vi "ex_subFileRead.vi"(0 "file path in":path, 1 "First Column is Time Channel":bool, 2 "file dialog?":bool, 3 "relative time?":bool, 4 "Attempt to Read Generic Text Files":bool, 5 "samples to read":i32=1, 6 "error in (no error)":errorcluster, 7 "delimiter":string="\t", 8 "First Row is Channel Names":bool, 9 "Decimal point":enum32{". (dot)", ", (comma)"}(radio), 10 "static path in":path, 11 "override samples":bool, 13 "Enable":bool=TRUE, 14 "Start Row":i32=1, 15 "storage_format":T6, 18 "single values":bool, 19 "Lock file":bool, 21 "Reset":bool) -> (12 "Description":string, 16 "Comment":string, 17 "EOF?":bool, 20 "file path out":path, 22 "Signals":dynamicdata(waveform), 26 "error out":errorcluster)   [LabVIEW 2020]
uses:
  <vilib>/express/express input/ExFileReadBlock.llb/ex_ReadFileGenericParams.ctl
  <vilib>/express/express shared/ExFile.llb/ex_FileFormats.ctl
  <vilib>/Platform/express/TDMExpress.llb/ex_readInfoTDM.ctl
  <vilib>/Platform/express/TDMExpress.llb/ex_readChannelInfo.ctl
  <vilib>/express/express shared/ExFile.llb/ex_TdmData.ctl
  <vilib>/express/express shared/ExFile.llb/ex_TdmProperty.ctl
  <vilib>/express/express shared/ex_EditUserDefinedProperties/usiDataType.ctl
panel:
  in  "Boolean":bool
  in  "read info":T1
  in  "read info in":T1
  in  "Lock file 2":bool
  out "previous path":path
  in  "Generic Params":T7
  in  "1st":bool
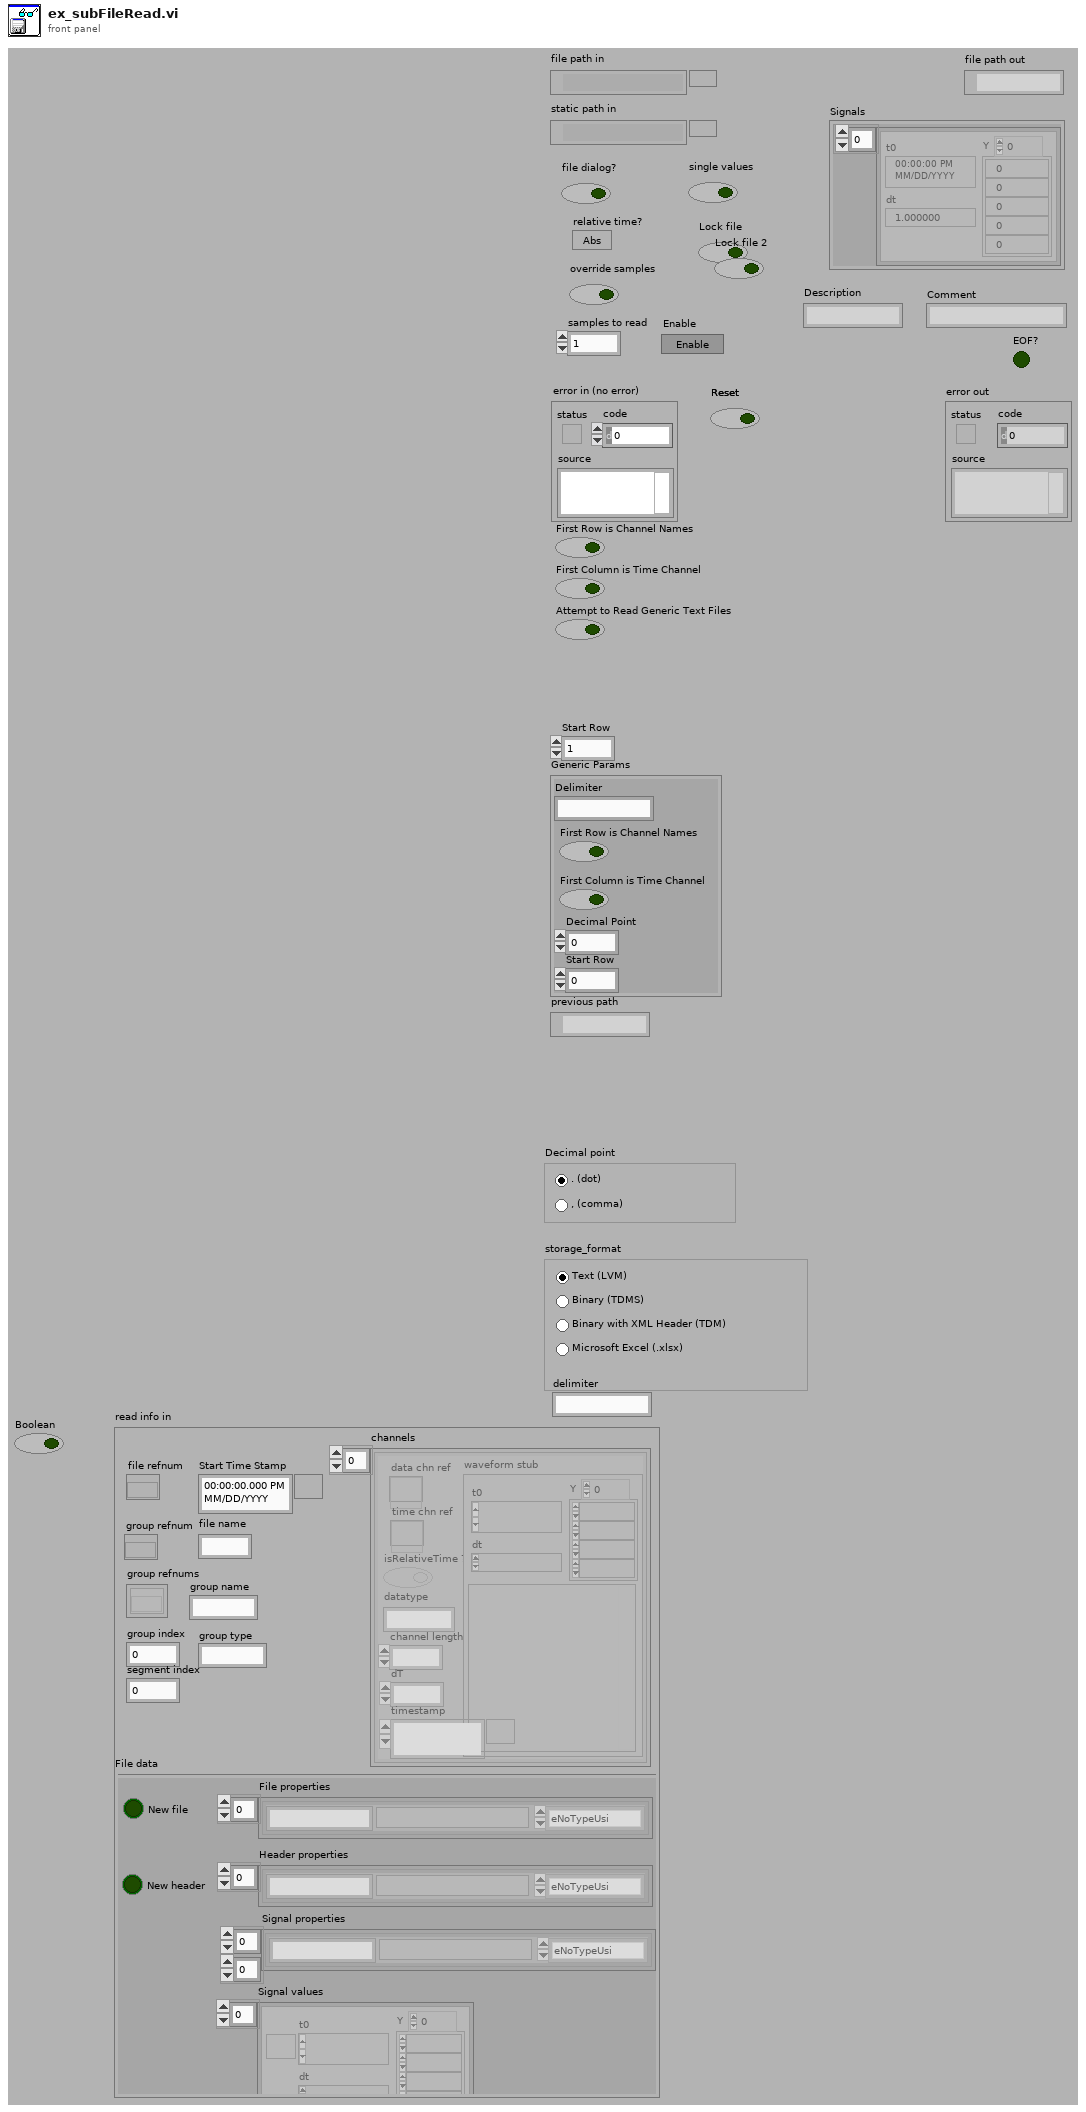
[diagram p1: front panel]
types:
  T1 = typedef "ex_readInfoTDM.ctl" = cluster{"file refnum":refnum<k20>, "group refnum":refnum<k20>, "group name":string, "group type":string, "Start Time Stamp":timestamp, "group index":u32, "group refnums":refnum<k20>[], "file name":string, "segment index":u32, "channels":T2[], "File data":T3}
  T2 = typedef "ex_readChannelInfo.ctl" = cluster{"data chn ref":refnum<k20>, "time chn ref":refnum<k20>, "isRelativeTime ?":bool, "channel length":u32, "dT":dbl, "waveform stub":waveform(dbl), "datatype":string, "timestamp":timestamp}
  T3 = typedef "ex_TdmData.ctl" = cluster{"New file":bool, "New header":bool, "File properties":T4[], "Header properties":T4[], "Signal properties":T4[][], "Signal values":waveform(dbl)[]}
  T4 = typedef "ex_TdmProperty.ctl" = cluster{"Name":string, "Type":T5, "Value":variant}
  T5 = typedef "usiDataType.ctl" = enum16{"eNoTypeUsi", "eInt8Usi", "eInt16Usi", "eInt32Usi", "eInt64Usi", "eUInt8Usi", "eUInt16Usi", "eUInt32Usi", "eUInt64Usi", "eFloat32Usi", "eFloat64Usi", "- 0", "- 1", "- 2", "- 3", "- 4", "- 5", "- 6", "- 7", "- 8", "- 9", "eString8Usi", "eString16Usi", "eStringUsi", "eEnumUsi", "- 10", "- 11", "- 12", "- 13", "- 14", "eTimeUsi", "- 15", "- 16", "- 17", "- 18", "- 19", "- 20", "- 21", "- 22", "- 23", "eInstanceUsi", "eStoreUsi"}
  T6 = typedef "ex_FileFormats.ctl" = enum32{"lvm", "tdm", "tdms", "xlsx"}
  T7 = typedef "ex_ReadFileGenericParams.ctl" = cluster{"Delimiter":string, "First Row is Channel Names":bool, "First Column is Time Channel":bool, "Decimal Point":i32, "Start Row":i32}
  T8 = typedef "ex_ReadFileParams.ctl" = cluster{"include col headings?":bool, "x_columns":u16, "col headings always?":bool, "time preference":u16, "hide col headings":bool}
  T9 = typedef "ex_AllChanInfo.ctl" = cluster{"No.Samples":i32, "Timestamp":timestamp, "X Dimension":string, "Y Dimension":string, "X0":timestamp, "Delta X":dbl, "Signal Name":string, "X Unit Label":string, "Y Unit Label":string}
  T10 = typedef "ex_FileReference.ctl" = cluster{"file ref":refnum<file>, "file size (bytes:0)":i32, "read pointer (bytes:0)":i32, "chunk size (bytes:65000)":i32}
  T11 = cluster{"chunk in":string, "file_params":T8, "delimiter":string, "optional info":cluster{"description":string, "operator":string, "project":string}, "Generic Header In":string[], "channel info":T9[], "read segment header in":bool, "# of samples read (in)":u32, "# of samples to read":i32, "# of samples in Channel Group":i32, "file refs in":T10, "origin timestamp":timestamp, "Is generic text file":bool, "Decimal Separator":string}
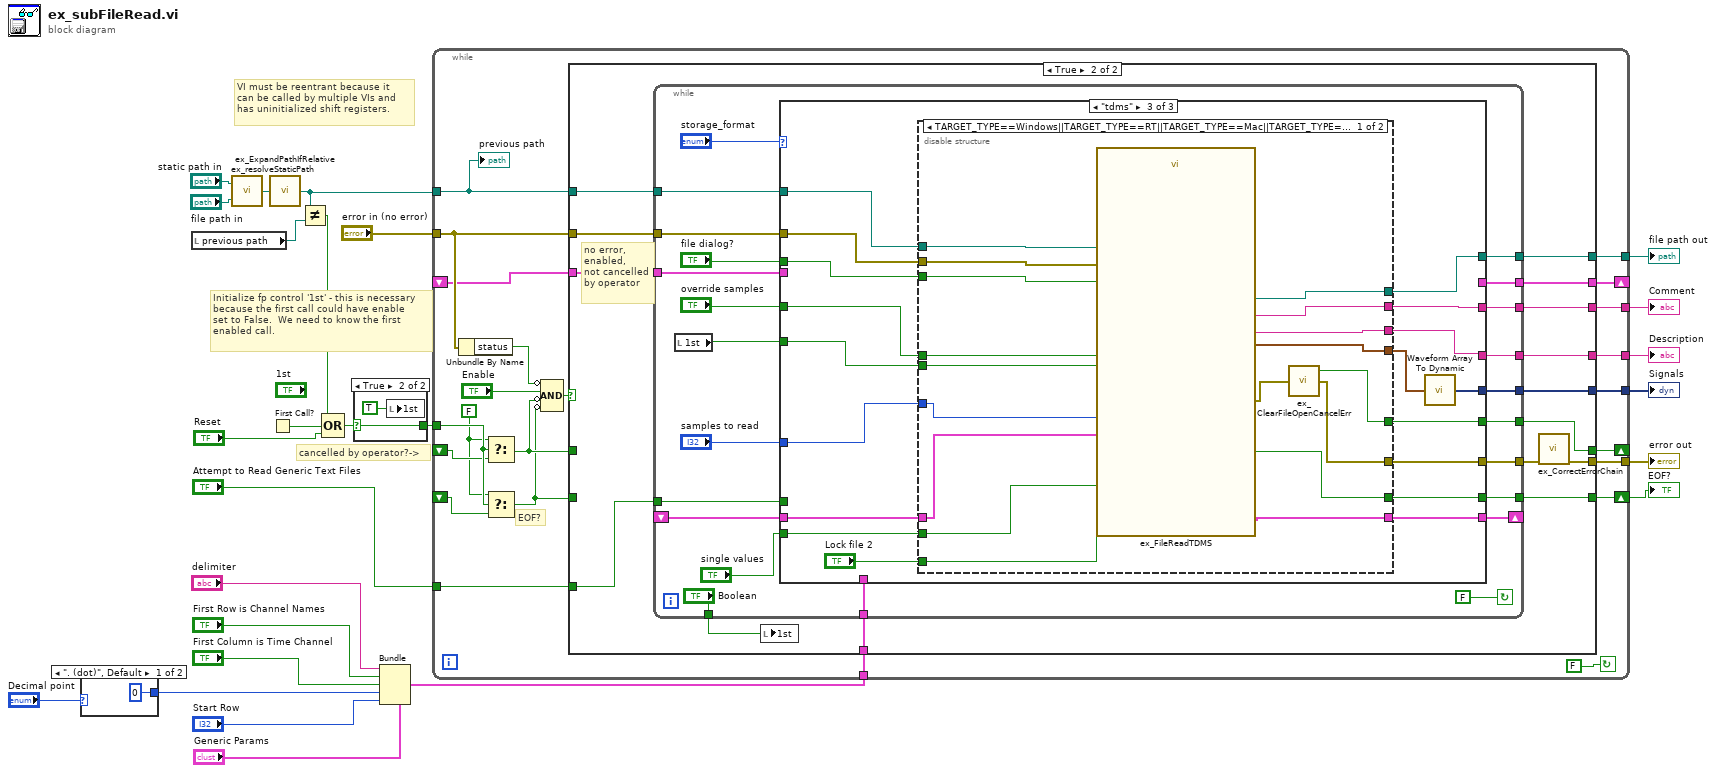
[diagram p0: block diagram]
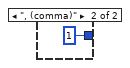
[diagram p2: hidden frame]
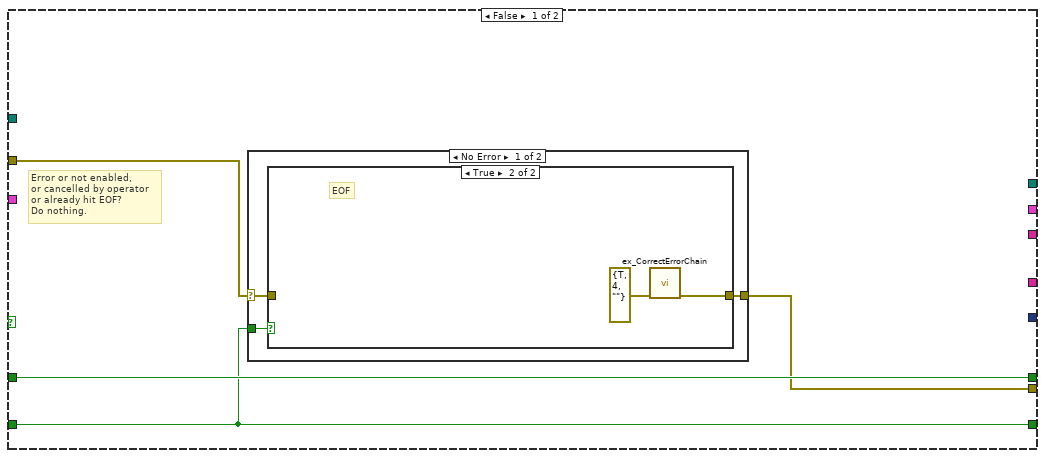
[diagram p3: hidden frame]
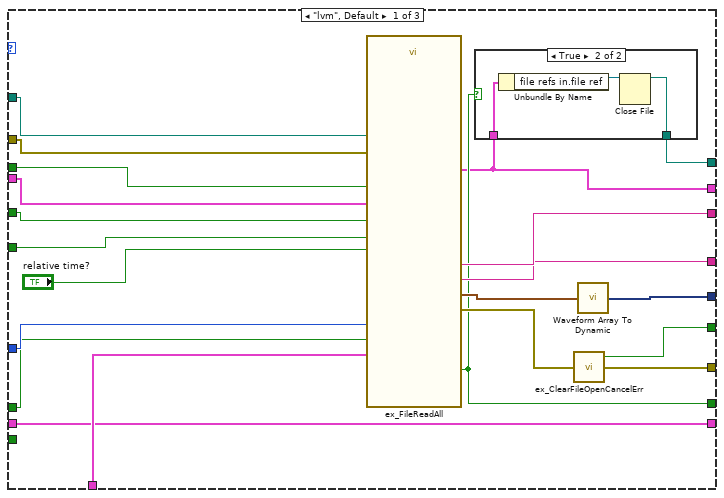
[diagram p6: hidden frame]
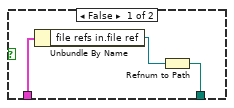
[diagram p7: hidden frame]
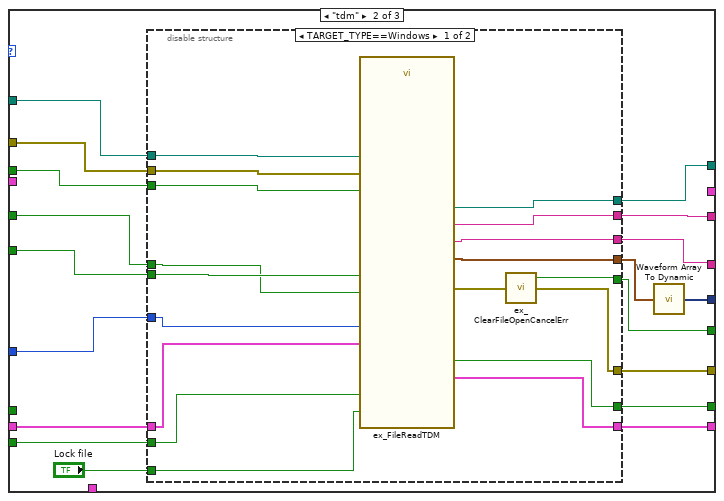
[diagram p8: hidden frame]
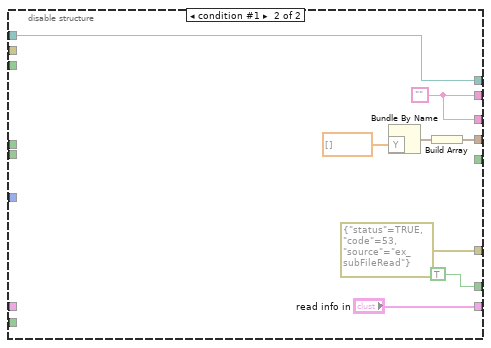
[diagram p9: hidden frame]
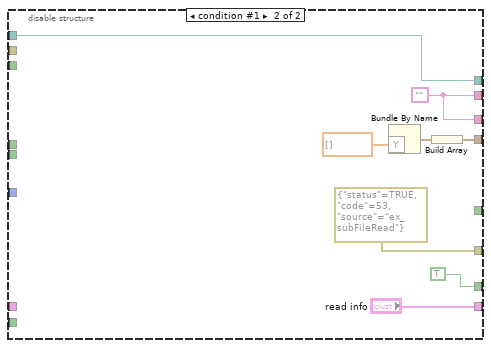
[diagram p10: hidden frame]
diagram:
  # "cancelled by operator?->"
  # "Initialize fp control '1st' - this is necessary \nbecause the first call could have enable \nset to False.  We need to know the first\nenabled call."
  # "VI must be reentrant because it \ncan be called by multiple VIs and \nhas uninitialized shift registers."
  n1 = case shown="\". (dot)\", Default" "Decimal point" {
    tunnel: [0 1] -> w3
    frame ". (dot)", Default {
    }
    frame ", (comma)" {
    }
  }
  n2 = local read "previous path"() -> (w14:path)
  n3 = call <vilib>:"ex_resolveStaticPath.vi"("file path in"="file path in", "static path in"="static path in") -> ("Path"=w15:path)
  n4 = First Call?() -> (First Call?: T/F=w26:bool)
  n5 = call <vilib>:"ex_ExpandPathIfRelative.vi"("Path"=w15) -> ("Expanded path"=w2:path)  [unwired: 4 out]
  n6 = Not Equal?(x=w2, y=w14) -> (x != y?=w12:bool)
  n7 = Compound Arithmetic op=OR(w12, w26, "Reset") -> (w13:bool)
  n8 = case shown="True" w13 {
    selector: w13 -> [w29 w30]
    tunnel: [w29 w30] -> w25
    frame False {
    }
    frame True {
      n9 = local write "1st"(TRUE ("1st")) -> ()
    }
  }
  n10 = Bundle(cluster="Generic Params", "Delimiter"="delimiter", "First Row is Channel Names"="First Row is Channel Names", "First Column is Time Channel"="First Column is Time Channel", "Decimal Point"=w3, "Start Row"="Start Row") -> (w18:T7)
  n11 = while {
    tunnel: [w54] -> w11
    tunnel: w25 -> [w40]
    tunnel: "error in (no error)" -> [w53]
    shift-right: [w49] -> _
    shift-left: _ -> [w39]
    tunnel: "Attempt to Read Generic Text Files" -> [w48]
    tunnel: w18 -> [w47]
    tunnel: w2 -> [w46]
    tunnel: [w45] -> w10
    tunnel: [w44] -> w9
    tunnel: [w43] -> w8
    tunnel: [w42] -> w7
    shift-right: [w41] -> w6
    shift-left: _ -> [w37]
    shift-right: [w32] -> _
    shift-left: _ -> [w33]
    stop <- FALSE continue-if-true
    w38 = FALSE ("operator cancelled?")
    # "EOF?"
    n12 = Unbundle By Name(w53) -> ("status"=w35:bool)
    n13 = Select(t=w38, s=w40, f=w39) -> (s? t:f=w36:bool)
    n14 = Select(t=w38, s=w40, f=w37) -> (s? t:f=w34:bool)
    n15 = Compound Arithmetic op=AND(invert w35, "Enable", invert w36, invert w34) -> (w50:bool)
    n16 = case shown="True" w50 {
      tunnel: [w56 w73] -> w54
      tunnel: w53 -> [w57 w80]
      tunnel: [w58 w78] -> w49
      tunnel: w36 -> [w58 _]
      tunnel: w48 -> [_ w77]
      tunnel: w47 -> [_ w76]
      tunnel: w46 -> [_ w75]
      tunnel: [_ w72] -> w45
      tunnel: [_ w71] -> w44
      tunnel: [_ w70] -> w43
      tunnel: [_ w69] -> w42
      tunnel: [w55 w68] -> w41
      tunnel: w34 -> [w55 _]
      tunnel: w33 -> [_ w67]
      tunnel: [_ w66] -> w32
      frame False {
        # "Error or not enabled,\nor cancelled by operator\nor already hit EOF?\nDo nothing."
        n17 = case shown="No Error" w57 {
          selector: w57 -> [w59 w65]
          tunnel: [w60 w65] -> w56
          tunnel: w55 -> [w61 _]
          frame No Error {
            n18 = case shown="True" w61 {
              tunnel: [w62 w64] -> w60
              tunnel: w59 -> [w62 _]
              frame False {
                # "not EOF"
              }
              frame True {
                # "EOF"
                n19 = call <vilib>:"ex_CorrectErrorChain.vi"("error in (no error)"=errorcluster {"status"=TRUE, "code"=4, "source"=""}) -> ("error out"=w64:errorcluster)  [unwired: 1 in, 9 out]
              }
            }
          }
          frame Error {
          }
        }
      }
      frame True {
        # "no error,\nenabled,\nnot cancelled\nby operator"
        n20 = while {
          tunnel: [w100] -> w74
          tunnel: w80 -> [w103]
          tunnel: ["Boolean"] -> w79
          tunnel: [w99] -> w78
          tunnel: w77 -> [w98]
          tunnel: w76 -> [w97]
          tunnel: w75 -> [w96]
          tunnel: [w95] -> w72
          tunnel: [w94] -> w71
          tunnel: [w93] -> w70
          tunnel: [w92] -> w69
          tunnel: [w91] -> w68
          tunnel: w67 -> [w86]
          tunnel: [w85] -> w66
          shift-right: [w82] -> _
          shift-left: _ -> [w83]
          stop <- FALSE continue-if-true
          n21 = local read "1st"() -> (w89:bool)
          n22 = case shown="\"tdms\"" "storage_format" {
            tunnel: w103 -> [w120 w147 w191]
            tunnel: [w124 w142 w186] -> w100
            tunnel: [w123 w131 w175] -> w99
            tunnel: w98 -> [w115 _ _]
            tunnel: w97 -> [w110 _ _]
            tunnel: w96 -> [w121 w148 w192]
            tunnel: [w105 w145 w189] -> w95
            tunnel: [w112 w144 w188] -> w94
            tunnel: [w111 w143 w187] -> w93
            tunnel: [w122 w133 w177] -> w92
            tunnel: [w107 w140 w184] -> w91
            tunnel: w89 -> [w118 w137 w181]
            tunnel: "samples to read" -> [w116 w141 w185]
            tunnel: "override samples" -> [w119 w136 w180]
            tunnel: w86 -> [w109 _ _]
            tunnel: [w106 _ _] -> w85
            tunnel: "file dialog?" -> [w108 w146 w190]
            tunnel: w83 -> [w104 w139 w183]
            tunnel: [w104 w138 w182] -> w82
            tunnel: "single values" -> [_ w135 w179]
            frame "lvm", Default {
              n23 = call <vilib>:"ex_FileReadAll.vi"("Parsing Data and Options In"=w109, "Generic File Read Parameters"=w110, "Attempt to Read Generic Text Files"=w115, "first_time?"=w118, "file dialog?"=w108, "error in (no error)"=w120, "file path in"=w121, "use specified sample size"=w119, "Samples to read"=w116, "relative time?"="relative time?") -> ("end-of-file?"=w107:bool, "Parsing Data and Options Out"=w106:T11, "Signals"=w113:waveform(dbl)[], "Description"=w111:string, "Comment"=w112:string, "error out"=w114:errorcluster)  [unwired: 4 out]
              n24 = case shown="True" w107 {
                tunnel: w106 -> [w127 w130]
                tunnel: [w126 w128] -> w105
                frame False {
                  n25 = Unbundle By Name(w127) -> ("file refs in.file ref"=w125:refnum<file>)
                  n26 = Refnum to Path(1:w125) -> (0:w126:path)
                }
                frame True {
                  n27 = Unbundle By Name(w130) -> ("file refs in.file ref"=w129:refnum<file>)
                  n28 = Close File(refnum=w129) -> (path=w128:path)  [unwired: 1 in, 1 out]
                }
              }
              n29 = call <vilib>:"ex_ClearFileOpenCancelErr.vi"("error in"=w114) -> ("error out"=w124:errorcluster, "cancelled?"=w123:bool)  [unwired: 3 out]
              n30 = call <vilib>:"Waveform Array To Dynamic.vi"("Input"=w113) -> ("Output"=w122:dynamicdata)  [unwired: 4 out]
            }
            frame "tdm" {
              n31 = disable-structure shown="TARGET_TYPE==Windows" {
                disable-tunnel: w148 -> [w166 w174]
                disable-tunnel: w147 -> [w152 _]
                disable-tunnel: w146 -> [w165 _]
                disable-tunnel: [w164 w174] -> w145
                disable-tunnel: [w163 w172] -> w144
                disable-tunnel: [w162 w172] -> w143
                disable-tunnel: [w150 errorcluster {"status"=TRUE, "code"=53, "source"="ex_subFileRead"} ("error in (no error)")] -> w142
                disable-tunnel: w141 -> [w161 _]
                disable-tunnel: [w160 TRUE ("EOF")] -> w140
                disable-tunnel: w139 -> [w153 _]
                disable-tunnel: [w159 "read info in"] -> w138
                disable-tunnel: w137 -> [w158 _]
                disable-tunnel: w136 -> [w157 _]
                disable-tunnel: w135 -> [w156 _]
                disable-tunnel: "Lock file" -> [w155 _]
                disable-tunnel: [w154 w170] -> w132
                disable-tunnel: [w149 _] -> w131
                frame condition #0 (active) {
                  n32 = call <vilib>:"ex_FileReadTDM.vi"("file path in"=w166, "Read specified segment size"=w157, "First time?"=w158, "Ask user for file"=w165, "Segment Size"=w161, "error in (no error)"=w152, "read info in"=w153, "single values"=w156, "Lock file"=w155) -> ("read info out"=w159:T1, "file path out"=w164:path, "Comment"=w163:string, "Signals"=w154:waveform(dbl)[], "Description"=w162:string, "EOF"=w160:bool, "error out"=w151:errorcluster)  [unwired: 1 in, 3 out]
                  n33 = call <vilib>:"ex_ClearFileOpenCancelErr.vi"("error in"=w151) -> ("error out"=w150:errorcluster, "cancelled?"=w149:bool)  [unwired: 3 out]
                }
                frame condition #1 {
                  w172 = ""
                  n34 = Bundle By Name("Y"=dbl[] []) -> (w171:waveform(dbl))  [unwired: 1 in]
                  n35 = Build Array(w171) -> (w170:waveform(dbl)[])
                }
              }
              n36 = call <vilib>:"Waveform Array To Dynamic.vi"("Input"=w132) -> ("Output"=w133:dynamicdata)  [unwired: 4 out]
            }
            frame "tdms" {
              n37 = disable-structure shown="TARGET_TYPE==Windows||TARGET_TYPE==RT||TARGET_TYPE==Mac||TARGET_TYPE==Unix" {
                disable-tunnel: w192 -> [w210 w218]
                disable-tunnel: w191 -> [w209 _]
                disable-tunnel: w190 -> [w208 _]
                disable-tunnel: [w207 w218] -> w189
                disable-tunnel: [w206 w216] -> w188
                disable-tunnel: [w205 w216] -> w187
                disable-tunnel: [w194 errorcluster {"status"=TRUE, "code"=53, "source"="ex_subFileRead"} ("error in (no error)")] -> w186
                disable-tunnel: w185 -> [w204 _]
                disable-tunnel: [w203 TRUE ("EOF")] -> w184
                disable-tunnel: w183 -> [w196 _]
                disable-tunnel: [w202 "read info"] -> w182
                disable-tunnel: w181 -> [w201 _]
                disable-tunnel: w180 -> [w200 _]
                disable-tunnel: w179 -> [w199 _]
                disable-tunnel: "Lock file 2" -> [w198 _]
                disable-tunnel: [w197 w214] -> w176
                disable-tunnel: [w193 _] -> w175
                frame condition #0 (active) {
                  n38 = call <vilib>:"ex_FileReadTDMS.vi"("file path in"=w210, "Read specified segment size"=w200, "First time?"=w201, "Ask user for file"=w208, "Segment Size"=w204, "error in (no error)"=w209, "read info in"=w196, "single values"=w199, "Lock file"=w198) -> ("read info out"=w202:T1, "file path out"=w207:path, "Comment"=w206:string, "Signals"=w197:waveform(dbl)[], "Description"=w205:string, "EOF"=w203:bool, "error out"=w195:errorcluster)  [unwired: 2 in, 2 out]
                  n39 = call <vilib>:"ex_ClearFileOpenCancelErr.vi"("error in"=w195) -> ("error out"=w194:errorcluster, "cancelled?"=w193:bool)  [unwired: 3 out]
                }
                frame condition #1 {
                  w216 = ""
                  n40 = Bundle By Name("Y"=dbl[] []) -> (w215:waveform(dbl))  [unwired: 1 in]
                  n41 = Build Array(w215) -> (w214:waveform(dbl)[])
                }
              }
              n42 = call <vilib>:"Waveform Array To Dynamic.vi"("Input"=w176) -> ("Output"=w177:dynamicdata)  [unwired: 4 out]
            }
          }
        }
        n43 = local write "1st"(w79) -> ()
        n44 = call <vilib>:"ex_CorrectErrorChain.vi"("error in (no error)"=w74) -> ("error out"=w73:errorcluster)  [unwired: 1 in, 9 out]
      }
    }
    "previous path" <- w46
  }
  "error out" <- w11
  "Comment" <- w9
  "EOF?" <- w6
  "Description" <- w8
  "file path out" <- w10
  "Signals" <- w7
